vi "MergeValveRatios_PressureData.vi"(10 "New Calibration Refs":T1, 11 "Old Calibration Refs":T1) -> (1 "None already calibrated?":bool, 2 "Merged Calibration Refs":T1, 3 "Only New Calibration Refs":T1)   [LabVIEW 2016]
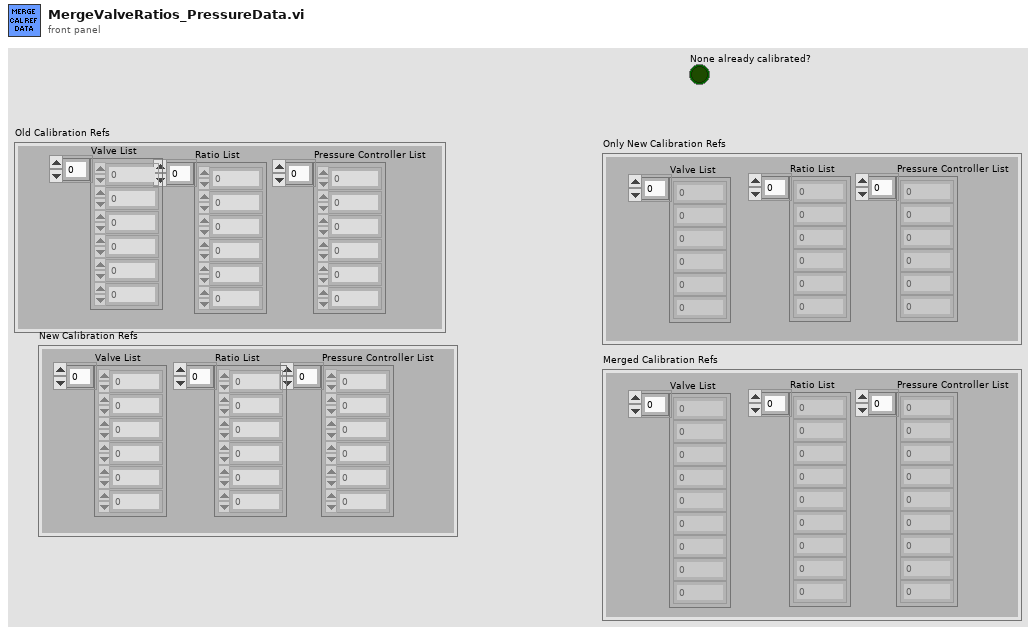
[diagram p1: front panel]
types:
  T1 = cluster{"Pressure Controller List":u8[], "Ratio List":dbl[], "Valve List":u16[]}
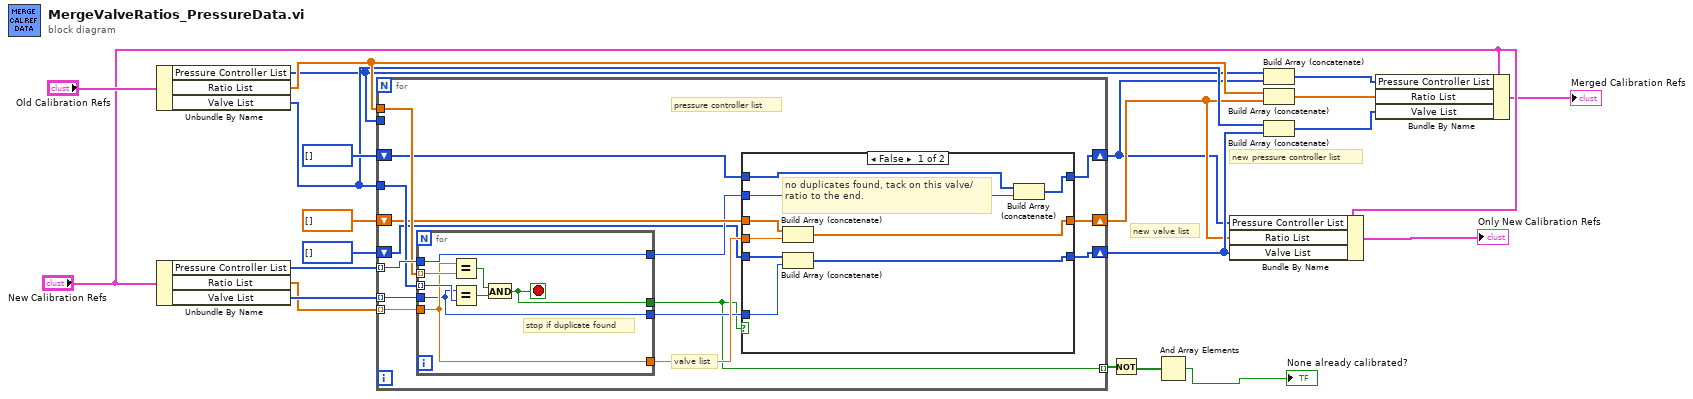
[diagram p0: block diagram]
diagram:
  # "new valve list"
  # "new pressure controller list"
  n1 = Unbundle By Name("Old Calibration Refs") -> ("Pressure Controller List"=w5:u8[], "Ratio List"=w15:dbl[], "Valve List"=w14:u16[])
  n2 = Unbundle By Name("New Calibration Refs") -> ("Pressure Controller List"=w19:u8[], "Ratio List"=w20:dbl[], "Valve List"=w21:u16[])
  n3 = for {
    tunnel: w14 -> [w34]
    tunnel: w15 -> [w33]
    tunnel: w5 -> [_]
    tunnel: w21 -> [w37] mode=indexing
    tunnel: w20 -> [w36] mode=indexing
    tunnel: w19 -> [w35] mode=indexing
    shift-right: [w31] -> w9
    shift-left: dbl[] [] -> [w30]
    shift-right: [w28] -> w4
    shift-left: u8[] [] -> [w27]
    shift-right: [w25] -> w10
    shift-left: u16[] [] -> [w24]
    tunnel: [w23] -> w3 mode=indexing
    # "pressure controller list"
    # "valve list"
    n4 = for {
      tunnel: w37 -> [w51]
      tunnel: w36 -> [w52]
      tunnel: w35 -> [w50]
      tunnel: w34 -> [w57] mode=indexing
      tunnel: w33 -> [w56] mode=indexing
      tunnel: [w53] -> w23
      tunnel: [w52] -> w32
      tunnel: [w51] -> w26
      tunnel: [w50] -> w29
      stop <- w53 stop-if-true
      # "stop if duplicate found"
      n5 = Equal?(x=w52, y=w56) -> (x = y?=w55:bool)
      n6 = Equal?(x=w51, y=w57) -> (x = y?=w54:bool)
      n7 = And(x=w55, y=w54) -> (x .and. y?=w53:bool)
    }
    n8 = case shown="False" w23 {
      tunnel: w32 -> [w46 _]
      tunnel: [w45 w49] -> w31
      tunnel: w30 -> [w44 w49]
      tunnel: w29 -> [w43 _]
      tunnel: [w42 w48] -> w28
      tunnel: w27 -> [w41 w48]
      tunnel: w26 -> [w40 _]
      tunnel: [w39 w47] -> w25
      tunnel: w24 -> [w38 w47]
      frame False {
        # "no duplicates found, tack on this valve/ratio to the end."
        n9 = Build Array (concatenate)(w44, w46) -> (w45:dbl[])
        n10 = Build Array (concatenate)(w38, w40) -> (w39:u16[])
        n11 = Build Array (concatenate)(w41, w43) -> (w42:u8[])
      }
      frame True {
        # "if a duplicate found, these data exist, so don't do anything"
      }
    }
  }
  n12 = Not(x=w3) -> (.not. x?=w2:bool[])
  n13 = And Array Elements(Boolean array=w2) -> (logical AND=→"None already calibrated?":bool)
  n14 = Bundle By Name(cluster="New Calibration Refs", "Pressure Controller List"=w4, "Ratio List"=w9, "Valve List"=w10) -> (→"Only New Calibration Refs":T1)
  n15 = Build Array (concatenate)(w5, w4) -> (w11:u8[])
  n16 = Build Array (concatenate)(w15, w9) -> (w12:dbl[])
  n17 = Build Array (concatenate)(w14, w10) -> (w13:u16[])
  n18 = Bundle By Name(cluster="New Calibration Refs", "Pressure Controller List"=w11, "Ratio List"=w12, "Valve List"=w13) -> (→"Merged Calibration Refs":T1)
